vi "line to strings.vi"(11 "line":T1) -> (3 "strings":string[](array[string]))   [LabVIEW 2015, in "Modbus Module editor node.lvclass"]
doc: "Platypus Framework 1.0.1.65\nNI Systems Engineering - National Instruments"
uses:
  Modbus Module editor node.lvclass
  table line.ctl
  module/module channel/Modbus Module Channel.lvclass
  <vilib>/NI/Tag Bus/tag/tag descriptor.lvclass/tag descriptor.ctl
  <vilib>/NI/Tag Bus Module Framework/channel/TBM channel.lvclass/TBM channel.ctl
  <vilib>/NI/Tag Bus/tag/read tag name.vi
  <vilib>/NI/Tag Bus Module Framework/channel/Read channel classification.vi
  <vilib>/NI/Tag Bus/tag/read data type.vi
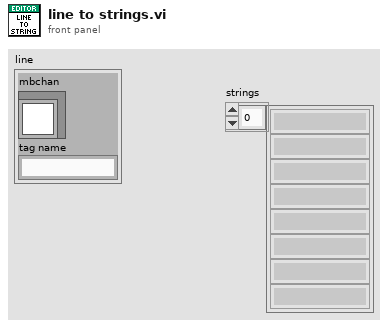
[diagram p1: front panel]
types:
  T1 = typedef "Modbus Module editor node.lvclass/table line.ctl" = cluster{"mbchan":refnum<class "Modbus Module Channel.lvclass">, "tag name":string}
  T2 = typedef "TBM channel.lvclass/channel classification.ctl" = enum16{"input data", "output data", "processing parameter", "processing result"}
  T3 = typedef "tag bus.lvlib/tag descriptor.lvclass/Data Type.ctl" = enum16{"Double", "Single", "I64", "I32", "I16", "I8", "U64", "U32", "U16", "U8", "Boolean", "String", "Array of Double", "Array of Single", "Array of I64", "Array of I32", "Array of I16", "Array of I8", "Array of U64", "Array of U32", "Array of U16", "Array of U8", "Array of Boolean", "Array of String"}
  T4 = typedef "Modbus Module editor node.lvclass/permissions.ctl" = enum32{"Read from MB", "Write to MB"}
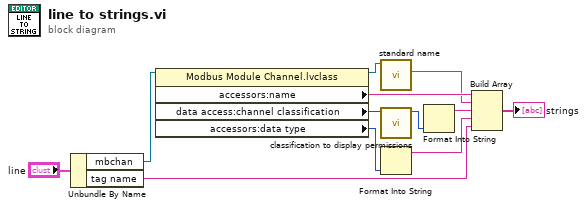
[diagram p0: block diagram]
diagram:
  n1 = Unbundle By Name("line") -> ("mbchan"=w6:refnum<class "Modbus Module Channel.lvclass">, "tag name"=w10:string)
  n2 = property class="Modbus Module Channel.lvclass"(reference=w6) -> (reference out=w2:refnum<class "Modbus Module Channel.lvclass">, "accessors:name"=w4:string, "data access:channel classification"=w5:T2, "accessors:data type"=w3:T3)  [unwired: 1 in, 1 out]
  n3 = call "standard name.vi"("Modbus Module Channel in"=w2) -> ("standard name"=w1:string)  [unwired: 8 in, 2 out]
  n4 = call "classification to display permissions.vi"("channel classification"=w5) -> ("permissions"=w8:T4)  [unwired: 10 in]
  n5 = Format Into String(w3) -> (resulting string=w11:string)  [unwired: 3 in, 1 out]
  n6 = Format Into String(w8) -> (resulting string=w7:string)  [unwired: 3 in, 1 out]
  n7 = Build Array(w4, w1, w7, w11, w10) -> (→"strings":string[])
